vi "solenoid_dual_okta.vi"(10 "INPUT_OKTA":bool, 11 "INPUT":bool) -> (2 "OUTPUT_B":bool, 3 "OUTPUT_A":bool)   [LabVIEW 2013]
panel:
  # "Dual Coil Solenoid with OK To Actuate:\n-If OKTA is Set, then OUTPUT A = INPUT and OUTPUT B = !INPUT. This drives a dual coil solenoid\n-If OKTA is clear, then OUTPUT A = 0 and OUTPUT B = 0. This is a 'safe' state."
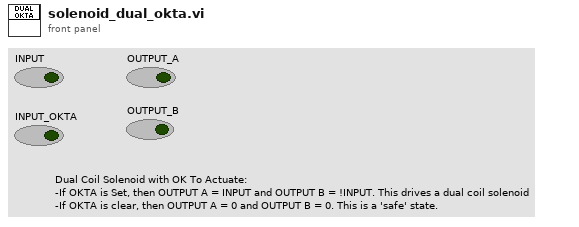
[diagram p1: front panel]
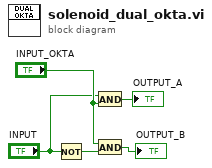
[diagram p0: block diagram]
diagram:
  n1 = Not(x="INPUT") -> (.not. x?=w4:bool)
  n2 = And(x="INPUT", y="INPUT_OKTA") -> (x .and. y?=→"OUTPUT_A":bool)
  n3 = And(x="INPUT_OKTA", y=w4) -> (x .and. y?=→"OUTPUT_B":bool)
